vi "subscribeToDataType.vi"(8 "error in":errorcluster, 9 "ObservableData":variant, 11 "ObserverClass in":refnum<class "ObserverClass.lvclass">) -> (0 "error out":errorcluster, 1 "ObservableValue":variant[](array[variant]), 2 "ObservableName":string[](array[string]), 3 "ObserverClass out":refnum<class "ObserverClass.lvclass">)   [LabVIEW 2025, in "ObserverClass.lvlib" / "ObserverClass.lvclass"]
doc: "Subscribe the Observable Data Type and Name for the current Observer Class istance.\nA List of Observable Name and Data Type can be obtained from a Cluster or a LV Class."
uses:
  ObserverClass.lvclass
  ObserverClass.lvclass/ObserverClass.ctl
  <vilib>/Utility/Data Type/NI_Data Type.lvlib
  <vilib>/PNR/LabVIEW Composition/Composition/Composition.lvlib
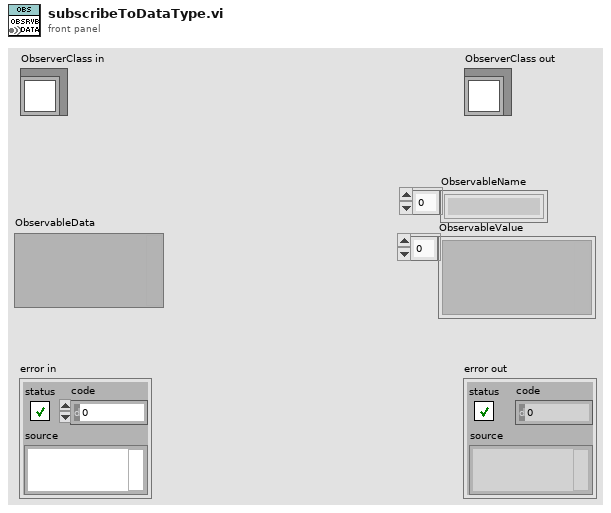
[diagram p1: front panel]
types:
  T1 = typedef "NI_Data Type.lvlib/Data Type.ctl" = enum8{"Invalid Type", "Void", "I8", "I16", "I32", "I64", "U8", "U16", "U32", "U64", "Single Float", "Double Float", "Extended Float", "Single Complex", "Double Complex", "Extended Complex", "Enum U8", "Enum U16", "Enum U32", "Enum U64", "Single Float With Unit", "Double Float With Unit", "Extended Float With Unit", "Single Complex with Unit", "Double Complex with Unit", "Extended Complex with Unit", "Boolean", "String", "Path", "Picture", "Tag", "Array", "Cluster", "Variant", "LV Variant", "Waveform", "Timestamp", "Digital Waveform", "Digital Data", "ExpressData", "Refnum", "External Data", "VI", "Poly VI", "LabVIEW Class Instance", "Fixed Point", "Set Collection", "Map Collection"}
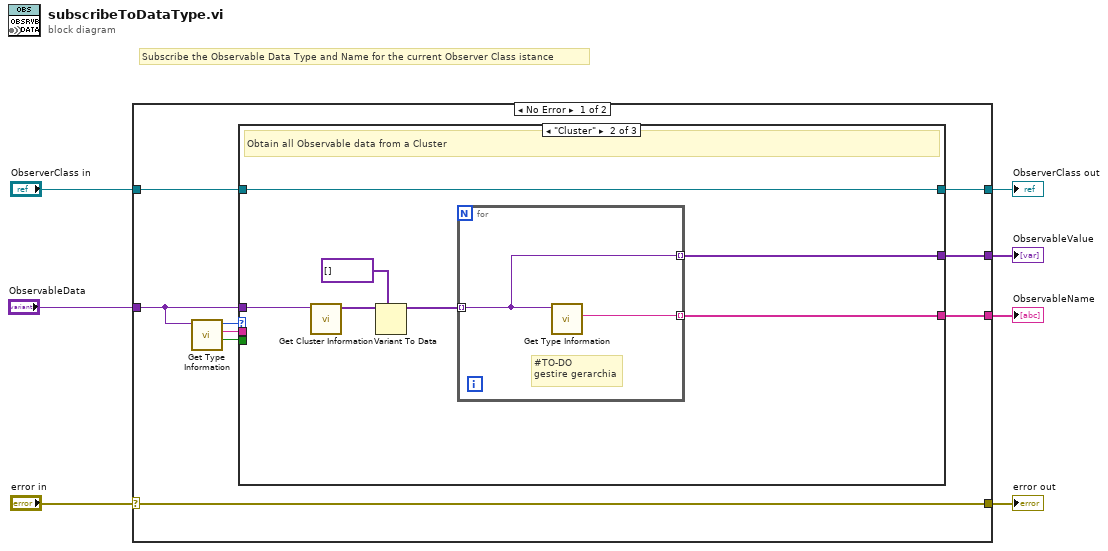
[diagram p0: block diagram]
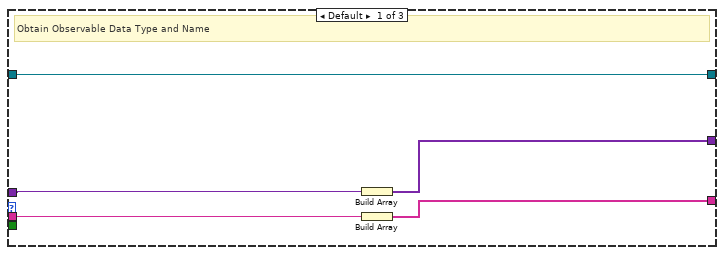
[diagram p2: hidden frame]
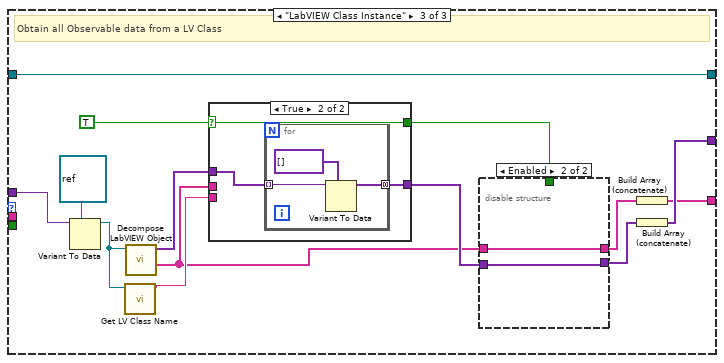
[diagram p3: hidden frame]
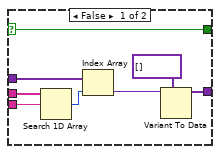
[diagram p5: hidden frame]
diagram:
  # "Subscribe the Observable Data Type and Name for the current Observer Class istance"
  n1 = case shown="No Error" "error in" {
    selector: "error in" -> [w16 w69]
    tunnel: [w16 w69] -> w6
    tunnel: [w8 w68] -> w4
    tunnel: "ObserverClass in" -> [w9 w68]
    tunnel: [w15 _] -> w3
    tunnel: [w14 _] -> w2
    tunnel: "ObservableData" -> [w12 _]
    frame No Error {
      n2 = call <vilib>:"Get Type Information.vi"("variant"=w12) -> ("type definition"=w13:bool, "name"=w10:string, "type"=w11:T1)  [unwired: 6 in, 2 out]
      n3 = case shown="\"Cluster\"" w11 {
        tunnel: [w18 w25 w31] -> w15
        tunnel: [w19 w24 w32] -> w14
        tunnel: w12 -> [w20 w23 w35]
        tunnel: w13 -> [_ _ _]
        tunnel: w10 -> [w21 _ _]
        tunnel: w9 -> [w17 w22 w44]
        tunnel: [w17 w22 w44] -> w8
        frame Default {
          # "Obtain Observable Data Type and Name"
          n4 = Build Array(w20) -> (w19:variant[])
          n5 = Build Array(w21) -> (w18:string[])
        }
        frame "Cluster" {
          # "Obtain all Observable data from a Cluster"
          n6 = call <vilib>:"Get Cluster Information.vi"("variant"=w23) -> ("cluster elements"=w28:variant[])  [unwired: 9 in, 1 out]
          n7 = Variant To Data(type=variant[] [], Variant=w28) -> (data=w26:variant[])  [unwired: 1 in, 1 out]
          n8 = for {
            tunnel: w26 -> [w29] mode=indexing
            tunnel: [w30] -> w25 mode=indexing
            tunnel: [w29] -> w24 mode=indexing
            # "#TO-DO\ngestire gerarchia"
            n9 = call <vilib>:"Get Type Information.vi"("variant"=w29) -> ("name"=w30:string)  [unwired: 6 in, 4 out]
          }
        }
        frame "LabVIEW Class Instance" {
          # "Obtain all Observable data from a LV Class"
          n10 = Variant To Data(type=refnum<class> refnum ("LabVIEW Object"), Variant=w35) -> (data=w39:refnum<class>)  [unwired: 1 in, 1 out]
          n11 = call <vilib>:"Get LV Class Name.vi"("object"=w39) -> ("class name"=w38:string)  [unwired: 9 in, 1 out]
          n12 = call <vilib>:"Decompose LabVIEW Object.vi"("LabVIEW Object"=w39) -> ("Class Names"=w33:string[], "Private Data Clusters"=w37:variant[])  [unwired: 7 in, 2 out]
          n13 = case shown="True" TRUE {
            selector: TRUE -> [w54 w62]
            tunnel: w37 -> [w59 w64]
            tunnel: [w61 w63] -> w42
            tunnel: w33 -> [w57 _]
            tunnel: w38 -> [w56 _]
            tunnel: [w54 w62] -> w36
            frame False {
              n14 = Search 1D Array(1D array=w57, element=w56) -> (index of element=w58:i32)  [unwired: 1 in]
              n15 = Index Array(array=w59, index=w58) -> (element=w60:variant)
              n16 = Variant To Data(type=variant[] [], Variant=w60) -> (data=w61:variant[])  [unwired: 1 in, 1 out]
            }
            frame True {
              n17 = for {
                tunnel: w64 -> [w66] mode=indexing
                tunnel: [w65] -> w63 mode=concatenating
                n18 = Variant To Data(type=variant[] [], Variant=w66) -> (data=w65:variant[])  [unwired: 1 in, 1 out]
              }
            }
          }
          n19 = disable-structure shown="Enabled" {
            disable-tunnel: w42 -> [w49 w52]
            disable-tunnel: [w48 w52] -> w41
            disable-tunnel: [w47 w53] -> w40
            disable-tunnel: w36 -> [w46 _]
            disable-tunnel: w33 -> [w45 w53]
            frame Disabled {
              n20 = for {
                tunnel: w49 -> [w51] mode=indexing
                tunnel: [w50] -> w47 mode=concatenating
                tunnel: [w51] -> w48 mode=concatenating
                tunnel: w46 -> [_]
                tunnel: w45 -> [w50] mode=indexing
              }
            }
            frame Enabled {
            }
          }
          n21 = Build Array (concatenate)(w40) -> (w31:string[])
          n22 = Build Array (concatenate)(w41) -> (w32:variant[])
        }
      }
    }
    frame Error {
    }
  }
  "error out" <- w6
  "ObserverClass out" <- w4
  "ObservableName" <- w3
  "ObservableValue" <- w2
